vi "Generic command handler.vi"(8 "error in (no error)":errorcluster, 10 "Message in":refnum<class "GenericMessage.lvclass">, 11 "LineCCD in":refnum<class "LineCCD.lvclass">) -> (0 "error out":errorcluster, 2 "value":string, 3 "LineCCD out":refnum<class "LineCCD.lvclass">)   [LabVIEW 2012, in "LineCCD.lvclass"]
doc: "The generic_command_handler processes the command 'generic'. Commands which are not part of the predefined list of commands fall under the 'generic' command for special activity."
uses:
  LineCCD.lvclass
  <vilib>/Distrio/Murmex/GenericMessage/GenericMessage.lvclass
  <vilib>/Distrio/Murmex/Murmex/Murmex.lvclass
  LineCCD.lvclass/LineCCD.ctl
  <vilib>/vision/NI_Vision_Development_Module.lvlib
panel:
  # "This method is called when the GENERIC\ntrigger is sent. \n\nOverride this method when your component needs to\nrespond to this trigger. \n\nCall parent for proper implementation"
  # "row"
  # "col"
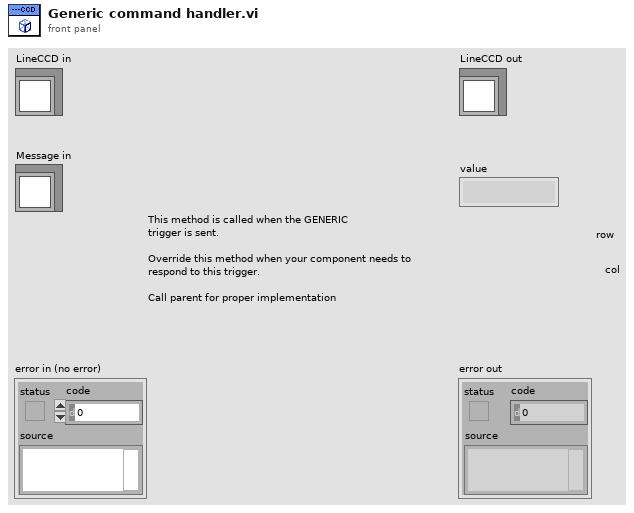
[diagram p1: front panel]
types:
  T1 = cluster{"y_min":refnum<vi>, "y_mean":refnum<vi>, "A_g":refnum<vi>, "STD":refnum<vi>, "x_0":refnum<vi>}
  T2 = typedef "LineCCD.lvclass/fitting parameters.ctl" = cluster{"y_min":dbl, "y_mean":dbl, "A_g":dbl, "STD":dbl, "x_0":dbl}
  T3 = typedef "IMAQ Image.ctl" = refnum<image>
  T4 = typedef "ROI Descriptor" = cluster{"Global Rectangle":i32[], "Contours":cluster{"ID":enum32{"External", "Internal"}, "Type":u32, "Coordinates":i32[]}[]}
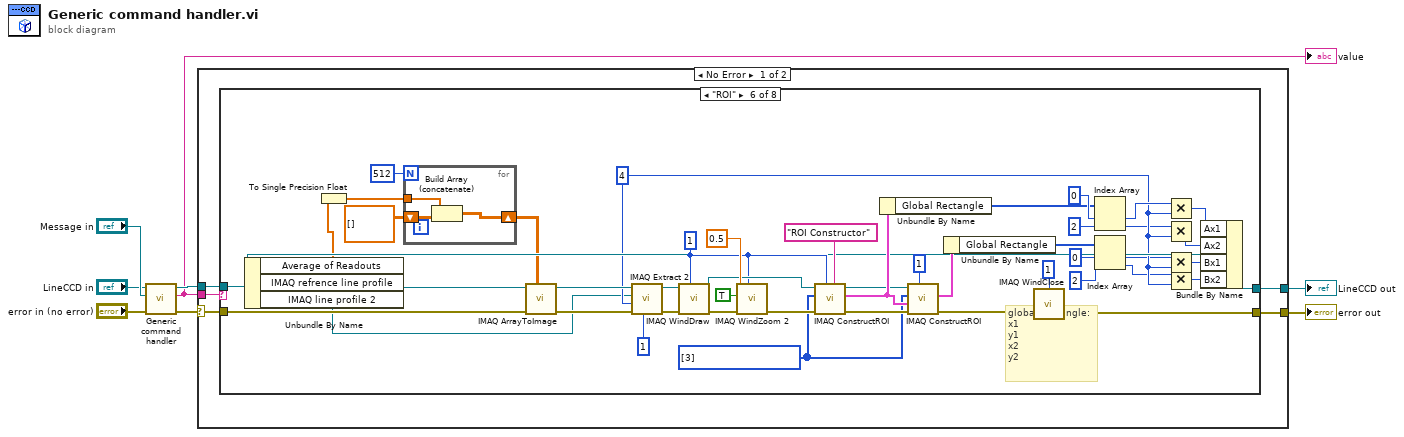
[diagram p0: block diagram]
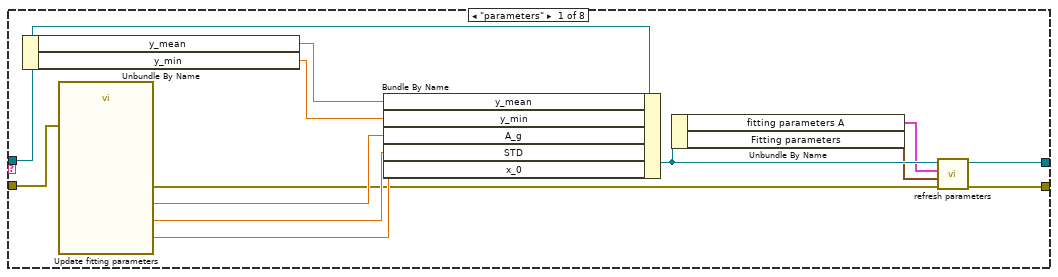
[diagram p2: hidden frame]
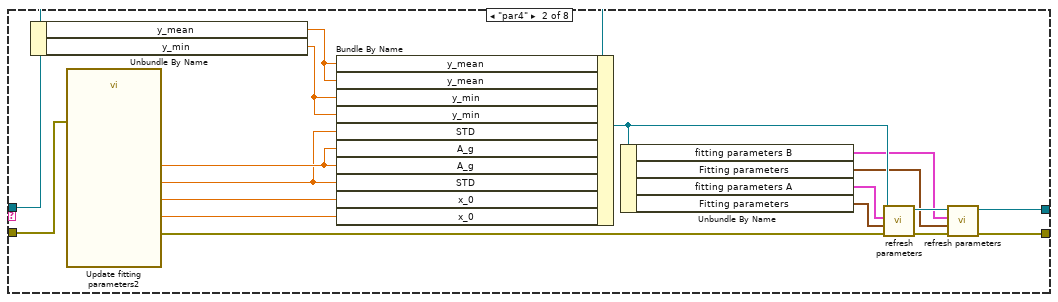
[diagram p3: hidden frame]
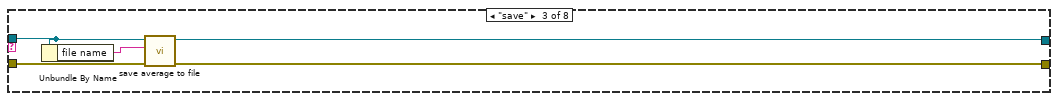
[diagram p4: hidden frame]
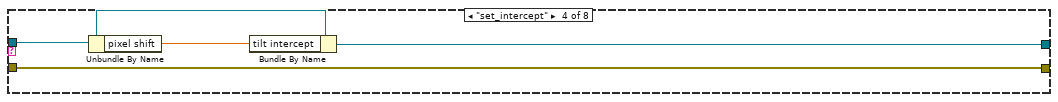
[diagram p5: hidden frame]
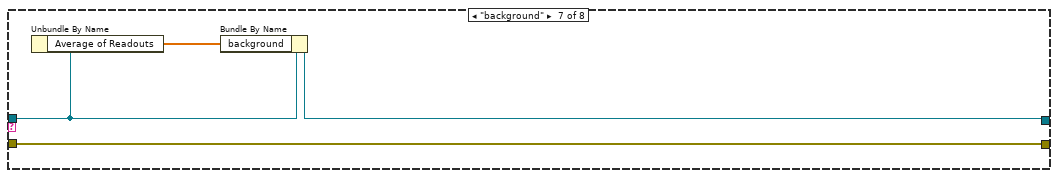
[diagram p7: hidden frame]
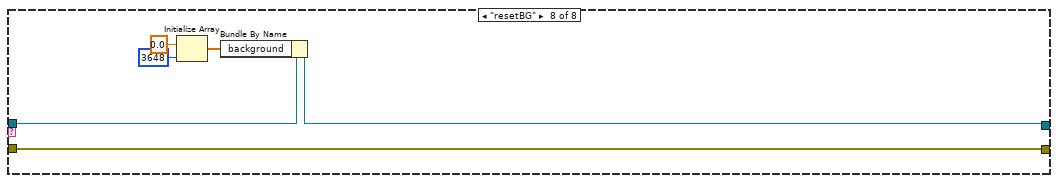
[diagram p8: hidden frame]
diagram:
  n1 = call-parent "Generic command handler.vi"("error in (no error)"="error in (no error)", "Message in"="Message in", "Murmex in"="LineCCD in") -> ("error out"=w5:errorcluster, "value"=w1:string, "Murmex out"=w4:refnum<class "LineCCD.lvclass">)  [unwired: 6 in]
  "value" <- w1
  n2 = case shown="No Error" w5 {
    selector: w5 -> [w12 w116]
    tunnel: w4 -> [w11 w115]
    tunnel: w1 -> [w13 _]
    tunnel: [w9 w116] -> w3
    tunnel: [w10 w115] -> w2
    frame No Error {
      n3 = case shown="\"ROI\"" w13 {
        tunnel: w12 -> [w26 w44 w49 w51 w55 w101 w108 w114]
        tunnel: w11 -> [w16 w33 w46 w53 w54 w78 w107 w113]
        tunnel: [w21 w32 w45 w50 w54 w77 w106 w112] -> w10
        tunnel: [w20 w31 w48 w51 w55 w87 w108 w114] -> w9
        frame "parameters" {
          n4 = Unbundle By Name(w16) -> ("y_mean"=w14:dbl, "y_min"=w15:dbl)
          n5 = call "Update fitting parameters"("error in (no error)"=w26) -> ("x_0"=w23:dbl, "STD"=w24:dbl, "A_g"=w25:dbl, "error out"=w22:errorcluster)  [unwired: 14 in, 1 out]
          n6 = Bundle By Name(cluster=w16, "y_mean"=w14, "y_min"=w15, "A_g"=w25, "STD"=w24, "x_0"=w23) -> (w19:refnum<class "LineCCD.lvclass">)
          n7 = Unbundle By Name(w19) -> ("fitting parameters A"=w17:T1, "Fitting parameters"=w18:T2)
          n8 = call-dynamic "refresh parameters.vi"("error in (no error)"=w22, "runtime.Fitting.FIT_A.Fitting parameters"=w18, "cluster"=w17, "LineCCD in"=w19) -> ("error out"=w20:errorcluster, "LineCCD out"=w21:refnum<class "LineCCD.lvclass">)  [unwired: 6 in]
        }
        frame "par4" {
          n9 = Unbundle By Name(w33) -> ("y_mean"=w27:dbl, "y_min"=w28:dbl)
          n10 = call "Update fitting parameters2"("error in (no error)"=w44) -> ("x_0_B"=w42:dbl, "x_0_A"=w43:dbl, "STD"=w29:dbl, "A_g"=w30:dbl, "error out"=w40:errorcluster)  [unwired: 13 in, 1 out]
          n11 = Bundle By Name(cluster=w33, "y_mean"=w27, "y_mean"=w27, "y_min"=w28, "y_min"=w28, "STD"=w29, "A_g"=w30, "A_g"=w30, "STD"=w29, "x_0"=w43, "x_0"=w42) -> (w38:refnum<class "LineCCD.lvclass">)
          n12 = Unbundle By Name(w38) -> ("fitting parameters B"=w34:T1, "Fitting parameters"=w35:T2, "fitting parameters A"=w36:T1, "Fitting parameters"=w37:T2)
          n13 = call-dynamic "refresh parameters.vi"("error in (no error)"=w40, "runtime.Fitting.FIT_A.Fitting parameters"=w37, "cluster"=w36, "LineCCD in"=w38) -> ("error out"=w41:errorcluster, "LineCCD out"=w39:refnum<class "LineCCD.lvclass">)  [unwired: 6 in]
          n14 = call-dynamic "refresh parameters.vi"("error in (no error)"=w41, "runtime.Fitting.FIT_A.Fitting parameters"=w35, "cluster"=w34, "LineCCD in"=w39) -> ("error out"=w31:errorcluster, "LineCCD out"=w32:refnum<class "LineCCD.lvclass">)  [unwired: 6 in]
        }
        frame "save" {
          n15 = Unbundle By Name(w46) -> ("file name"=w47:string)
          n16 = call-dynamic "save average to file.vi"("error in (no error)"=w49, "filename"=w47, "LineCCD in"=w46) -> ("error out"=w48:errorcluster, "LineCCD out"=w45:refnum<class "LineCCD.lvclass">)  [unwired: 7 in]
        }
        frame "set_intercept" {
          n17 = Unbundle By Name(w53) -> ("pixel shift"=w52:dbl)
          n18 = Bundle By Name(cluster=w53, "tilt intercept"=w52) -> (w50:refnum<class "LineCCD.lvclass">)
        }
        frame Default {
        }
        frame "ROI" {
          w66 = 4 ("X Step Size")
          w85 = u32[] [3] items=["No Selection", "Point", "Line", "Rectangle", "Oval", "Polygon", "Freehand Region", "Annulus", "Zoom", "Pan", "Broken Line", "Freehand Line", "Rotated Rectangle"] ("Tools")
          w97 = 1 ("Window Number (0...15)")
          # "global rectangle:\nx1\ny1\nx2\ny2"
          n19 = Unbundle By Name(w78) -> ("Average of Readouts"=w70:dbl[], "IMAQ refrence line profile"=w100:T3, "IMAQ line profile 2"=w57:T3)
          n20 = To Single Precision Float(number=w70) -> (single precision float=w69:sgl[])
          n21 = for {
            N: 512 -> [_]
            tunnel: w69 -> [w104]
            shift-right: [w103] -> w68
            shift-left: sgl[][] [] -> [w102]
            n22 = Build Array (concatenate)(w104, w102) -> (w103:sgl[][])
          }
          n23 = call "IMAQ ArrayToImage"("Image Pixels (Float)"=w68, "error in (no error)"=w101, "Image"=w100) -> ("error out"=w76:errorcluster, "Image Out"=w74:T3)  [unwired: 7 in]
          n24 = call "IMAQ Extract 2"("Y Step Size"=1, "error in (no error)"=w76, "X Step Size"=w66, "Image Dst"=w57, "Image Src"=w74) -> ("error out"=w75:errorcluster, "Image Dst Out"=w71:T3)  [unwired: 5 in]
          n25 = call "IMAQ WindDraw"("Window Number (0...15)"=w97, "error in (no error)"=w75, "Image"=w71) -> ("error out"=w94:errorcluster, "Image Out (duplicate)"=w98:T3)  [unwired: 7 in]
          n26 = call "IMAQ WindZoom 2"("Window Number (0...15)"=w97, "error in (no error)"=w94, "Zoom to Fit? (False)"=TRUE, "Zoom Factor"=sgl 0.5) -> ("error out"=w95:errorcluster)  [unwired: 4 in, 3 out]
          n27 = call "IMAQ ConstructROI"("Prompt"="ROI Constructor", "Window Number (-1...15)"=w97, "error in (no error)"=w95, "Tools"=w85, "Image"=w98) -> ("error out"=w91:errorcluster, "ROI Descriptor Out"=w90:T4, "Image Out (duplicate)"=w89:T3)  [unwired: 3 in, 1 out]
          n28 = Unbundle By Name(w90) -> ("Global Rectangle"=w81:i32[])
          n29 = call "IMAQ ConstructROI"("Window Number (-1...15)"=1, "error in (no error)"=w91, "ROI Descriptor In (None)"=w90, "Tools"=w85, "Image"=w89) -> ("error out"=w58:errorcluster, "ROI Descriptor Out"=w86:T4)  [unwired: 3 in, 2 out]
          n30 = Unbundle By Name(w86) -> ("Global Rectangle"=w80:i32[])
          n31 = call "IMAQ WindClose"("Window Number (0...15)"=1, "error in (no error)"=w58) -> ("error out"=w87:errorcluster)  [unwired: 4 in]
          n32 = Index Array(array=w81, index #1=0 ("index"), index #2=2 ("index")) -> (element #1=w67:i32, element #2=w65:i32)
          n33 = Index Array(array=w80, index #1=0 ("index"), index #2=2 ("index")) -> (element #1=w64:i32, element #2=w63:i32)
          n34 = Multiply(x=w67, y=w66) -> (x*y=w62:i32)
          n35 = Multiply(x=w65, y=w66) -> (x*y=w61:i32)
          n36 = Multiply(x=w64, y=w66) -> (x*y=w60:i32)
          n37 = Multiply(x=w63, y=w66) -> (x*y=w59:i32)
          n38 = Bundle By Name(cluster=w78, "Ax1"=w62, "Ax2"=w61, "Bx1"=w60, "Bx2"=w59) -> (w77:refnum<class "LineCCD.lvclass">)
        }
        frame "background" {
          n39 = Unbundle By Name(w107) -> ("Average of Readouts"=w105:dbl[])
          n40 = Bundle By Name(cluster=w107, "background"=w105) -> (w106:refnum<class "LineCCD.lvclass">)
        }
        frame "resetBG" {
          n41 = Initialize Array(0.0 ("element"), 3648 ("dimension size")) -> (w109:dbl[])
          n42 = Bundle By Name(cluster=w113, "background"=w109) -> (w112:refnum<class "LineCCD.lvclass">)
        }
      }
    }
    frame Error {
    }
  }
  "error out" <- w3
  "LineCCD out" <- w2
